vi "SetMaxPosition.vi"(8 "Error In":errorcluster, 10 "Max Position":dbl, 11 "Thorlabs In":refnum<class "Thorlabs.lvclass">) -> (0 "Error Out":errorcluster, 3 "Thorlabs Out":refnum<class "Thorlabs.lvclass">)   [LabVIEW 2018, in "Thorlabs.lvlib" / "Thorlabs.lvclass"]
doc: "This VI sets the Step Size on the job on the Axis.\n\nCreator: Slade Jeppesen\nCreated Date: 10/02/20"
uses:
  Thorlabs.lvclass
  Thorlabs.lvclass/Thorlabs.ctl
  C:/AME Test Engineering/LabVIEW/PPLs/Axis/DLLs/ThorLabs.MotionControl.KCube.DCServoCLI.dll
  PPLs/Axis/DLLs/ThorLabs.MotionControl.KCube.DCServoCLI.dll
  C:/AME Test Engineering/LabVIEW/PPLs/Axis/DLLs/Thorlabs.MotionControl.GenericMotorCLI.dll
  PPLs/Axis/DLLs/Thorlabs.MotionControl.GenericMotorCLI.dll
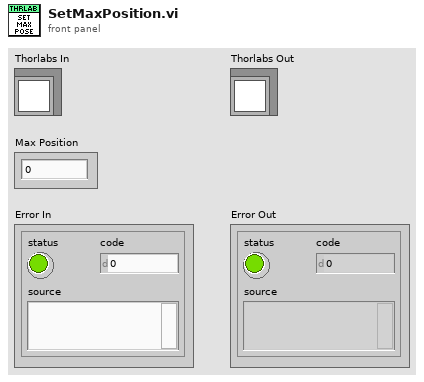
[diagram p1: front panel]
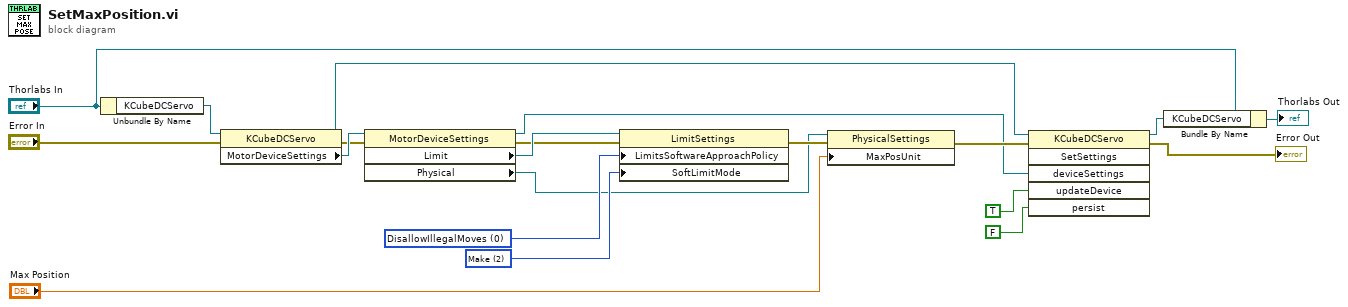
[diagram p0: block diagram]
diagram:
  w14 = 2 items=["Ignore"=1, "Make"=2, "Break"=3, "Home_Make"=4, "Home_Break"=5, "PMD_Index"=6, "Ignore_Swapped"=129, "Make_Swapped"=130, "Break_Swapped"=131, "Home_Make_Swapped"=132, "Home_Break_Swapped"=133] ("SoftLimitMode")
  w15 = i16 0 items=["DisallowIllegalMoves", "AllowPartialMoves", "AllowAllMoves"] ("LimitsSoftwareApproachPolicy")
  n1 = Unbundle By Name("Thorlabs In") -> ("KCubeDCServo"=w18:refnum<k24>)
  n2 = property class="KCubeDCServo"(reference=w18, error in="Error In") -> (reference out=w6:refnum<k24>, error out=w13:errorcluster, "MotorDeviceSettings"=w17:refnum<k24>)
  n3 = property class="MotorDeviceSettings"(reference=w17, error in=w13) -> (reference out=w3:refnum<k24>, error out=w12:errorcluster, "Limit"=w16:refnum<k24>, "Physical"=w10:refnum<k24>)
  n4 = property class="LimitSettings"(reference=w16, error in=w12, "LimitsSoftwareApproachPolicy"=w15, "SoftLimitMode"=w14) -> (error out=w11:errorcluster)  [unwired: 1 out]
  n5 = property class="PhysicalSettings"(reference=w10, error in=w11, "MaxPosUnit"="Max Position") -> (error out=w7:errorcluster)  [unwired: 1 out]
  n6 = invoke class="KCubeDCServo" method="SetSettings"(reference=w6, error in=w7, "deviceSettings"=w3, "updateDevice"=TRUE, "persist"=FALSE) -> (reference out=w8:refnum<k24>, error out=→"Error Out":errorcluster)  [unwired: 1 in, 4 out]
  n7 = Bundle By Name(cluster="Thorlabs In", "KCubeDCServo"=w8) -> (→"Thorlabs Out":refnum<class "Thorlabs.lvclass">)
